vi "NTJ_OldVer_Set_Persist.vi"(8 "error in (no error)":errorcluster, 10 "Persist Value":bool, 11 "Entry Name":string) -> (0 "error out":errorcluster)   [LabVIEW 2019]
uses:
  <vilib>/Rock Robotics/Network Tables/Create Actual Table Name.vi
  From_NTJ/NTJ_Build NT Field ID Buffer.vi
  <vilib>/Utility/error.llb/Clear Errors.vi
  <vilib>/Rock Robotics/Network Tables/NT Globals.vi
  <vilib>/Rock Robotics/Network Tables/Table Manager.vi
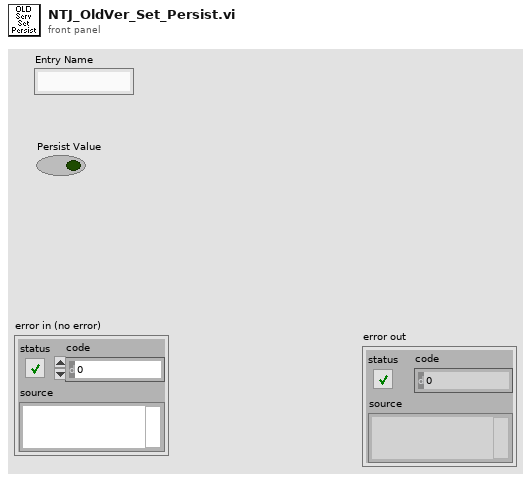
[diagram p1: front panel]
types:
  T1 = typedef "Field ID.ctl" = i32
  T2 = enum16{"Add Cnx", "Remove Cnx", "Retrieve List", "Cnx Inited"}
  T3 = enum16{"Update Field", "Read Field", "Assign Field", "Remove All", "Set Persistence", "Clear Persistence"}
  T4 = typedef "Field Data.ctl" = cluster{"Dbl":dbl, "String":string, "Type":T5, "Boolean":bool, "Sequence #":T6, "Flags":u8}
  T5 = typedef "Field Type.ctl" = enum8{"Invalid", "Bool", "Numeric", "String", "Raw", "Boolean Array", "Numeric Array", "String Array", "RPC"}
  T6 = typedef "Sequence.ctl" = u16
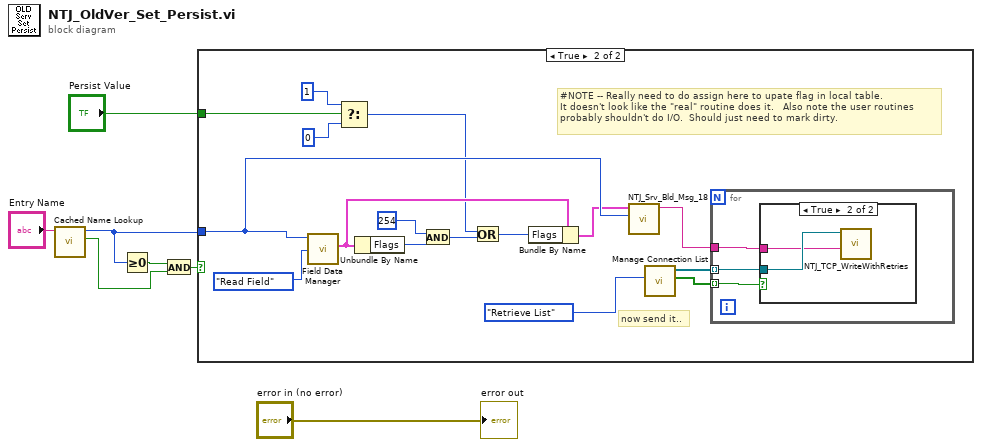
[diagram p0: block diagram]
diagram:
  n1 = call <vilib>:"Cached Name Lookup.vi"("Name"="Entry Name") -> ("Success"=w1:bool, "Entry ID"=w7:T1)  [unwired: 8 in, 1 out]
  n2 = Greater Or Equal To 0?(x=w7) -> (x >= 0?=w2:bool)
  n3 = And(x=w2, y=w1) -> (x .and. y?=w3:bool)
  n4 = case shown="True" w3 {
    tunnel: w7 -> [_ w19]
    tunnel: "Persist Value" -> [_ w9]
    frame False {
    }
    frame True {
      # "#NOTE -- Really need to do assign here to upate flag in local table.\nIt doesn't look like the \"real\" routine does it.   Also note the user routines\nprobably shouldn't do I/O.  Should just need to mark dirty."
      # "now send it.."
      n5 = call <vilib>:"Field Data Manager.vi"("Operation"=T3."Read Field", "Field ID"=w19) -> ("Field Value Out"=w17:T4)  [unwired: 8 in, 1 out]
      n6 = Select(t=u8 1, s=w9, f=u8 0 ("t")) -> (s? t:f=w12:u8)
      n7 = Unbundle By Name(w17) -> ("Flags"=w16:u8)
      n8 = And(x=u8 254, y=w16) -> (x .and. y?=w14:u8)
      n9 = Or(x=w12, y=w14) -> (x .or. y?=w13:u8)
      n10 = Bundle By Name(cluster=w17, "Flags"=w13) -> (w18:T4)
      n11 = call "NTJ_Srv_Bld_Msg_18.vi"("Field ID"=w19, "Field Value Out"=w18) -> ("Msg Buffer"=w20:string)  [unwired: 9 in]
      n12 = call <vilib>:"Manage Connection List.vi"("Operation"=T2."Retrieve List") -> ("Inited"=w8:bool[], "Connections List"=w21:refnum<k5>[])  [unwired: 8 in, 1 out]
      n13 = for {
        tunnel: w21 -> [w26] mode=indexing
        tunnel: w20 -> [w25]
        tunnel: w8 -> [w24] mode=indexing
        n14 = case shown="True" w24 {
          tunnel: w26 -> [_ w28]
          tunnel: w25 -> [_ w27]
          frame False {
          }
          frame True {
            n15 = call "NTJ_TCP_WriteWithRetries.vi"("Msg Buffer"=w27, "TCP Network Connection in"=w28) -> ()  [unwired: 8 in, 2 out]
          }
        }
      }
    }
  }
  "error out" <- "error in (no error)"
